vi "Initialize.vi"(7 "not in use":string="Setpoint.ch%d.SP", 8 "error in":errorcluster, 9 "Number of Channels":u32=1, 10 "Instance Name":string, 11 "Device in":refnum<class "Device.lvclass">) -> (0 "error out":errorcluster, 3 "Device out":refnum<class "Device.lvclass">)   [LabVIEW 2023, in "Device.lvclass"]
uses:
  Device.lvclass
  Device.lvclass/Device.ctl
  Low Level Capabilities/Current/Current Actual Value/Current Actual Value.lvclass
  Low Level Capabilities/Current/Current Setpoint/Current Setpoint.lvclass
  Low Level Capabilities/Voltage/Voltage Actual Value/Voltage Actual Value.lvclass
  Low Level Capabilities/Voltage/Voltage Setpoint/Voltage Setpoint.lvclass
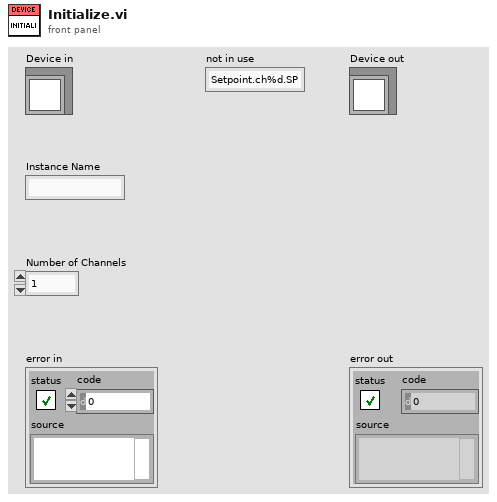
[diagram p1: front panel]
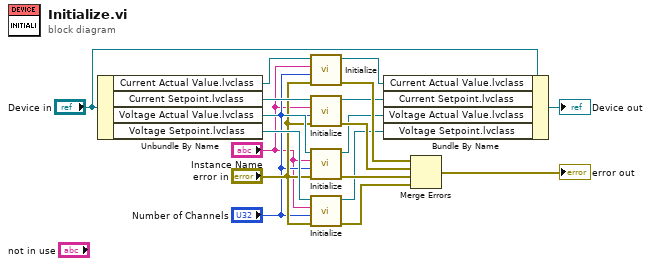
[diagram p0: block diagram]
diagram:
  n1 = Unbundle By Name("Device in") -> ("Current Actual Value.lvclass"=w18:refnum<class "Current Actual Value.lvclass">, "Current Setpoint.lvclass"=w17:refnum<class "Current Setpoint.lvclass">, "Voltage Actual Value.lvclass"=w9:refnum<class "Voltage Actual Value.lvclass">, "Voltage Setpoint.lvclass"=w8:refnum<class "Voltage Setpoint.lvclass">)
  n2 = call-dynamic "Initialize.vi"("error in"="error in", "Number of Channels"="Number of Channels", "Instance Name"="Instance Name", "Current Actual Value in"=w18) -> ("error out"=w15:errorcluster, "Current Actual Value out"=w11:refnum<class "Current Actual Value.lvclass">)  [unwired: 6 in]
  n3 = call-dynamic "Initialize.vi"("error in"="error in", "Number of Channels"="Number of Channels", "Instance Name"="Instance Name", "Current Setpoint in"=w17) -> ("error out 2"=w16:errorcluster, "Current Setpoint out"=w10:refnum<class "Current Setpoint.lvclass">)  [unwired: 6 in]
  n4 = call-dynamic "Initialize.vi"("error in"="error in", "Number of Channels"="Number of Channels", "Instance Name"="Instance Name", "Voltage Actual Value in"=w9) -> ("error out"=w14:errorcluster, "Voltage Actual Value out"=w6:refnum<class "Voltage Actual Value.lvclass">)  [unwired: 6 in]
  n5 = call-dynamic "Initialize.vi"("error in"="error in", "Number of Channels"="Number of Channels", "Instance Name"="Instance Name", "Voltage Setpoint in"=w8) -> ("error out 2"=w13:errorcluster, "Voltage Setpoint out"=w7:refnum<class "Voltage Setpoint.lvclass">)  [unwired: 6 in]
  n6 = Bundle By Name(cluster="Device in", "Current Actual Value.lvclass"=w11, "Current Setpoint.lvclass"=w10, "Voltage Actual Value.lvclass"=w6, "Voltage Setpoint.lvclass"=w7) -> (→"Device out":refnum<class "Device.lvclass">)
  n7 = Merge Errors(w15, w16, w14, w13) -> (→"error out":errorcluster)
